vi "Configure Multipoint.vi"(5 "Sample Interval (1 Second)":dbl=1.0 format="%#.6g", 6 "Sample Source (0: Immediate)":i32(ring) items=["Immediate", "Timer"], 7 "Pretrigger Count (0)":i32 format="%#.6g", 8 "error in (no error)":errorcluster, 9 "Sample Count (1)":i32=1 format="%#.6g", 10 "Trigger Count (1)":i32=1 format="%#.6g", 11 "VISA resource name":refnum<visa-resource-name>) -> (0 "error out":errorcluster, 3 "VISA resource name out":refnum<visa-resource-name>)   [LabVIEW 2020, in "Agilent 3446X Series.lvlib"]
doc: "Configures trigger count and sample count so you can take multipoint measurements.\n\nNote: Use this VI only with other low-level VIs. The high-level VIs automatically incorporate this functionality."
uses:
  Agilent 3446X Series.lvlib
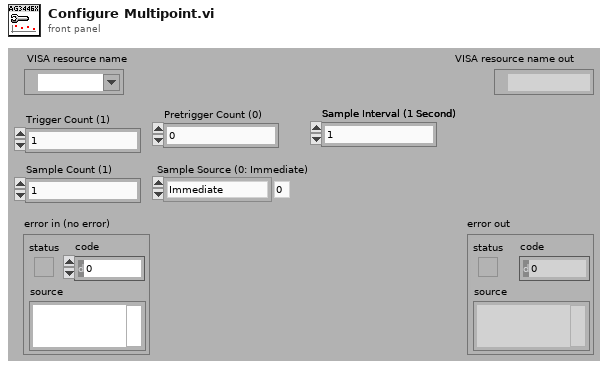
[diagram p1: front panel]
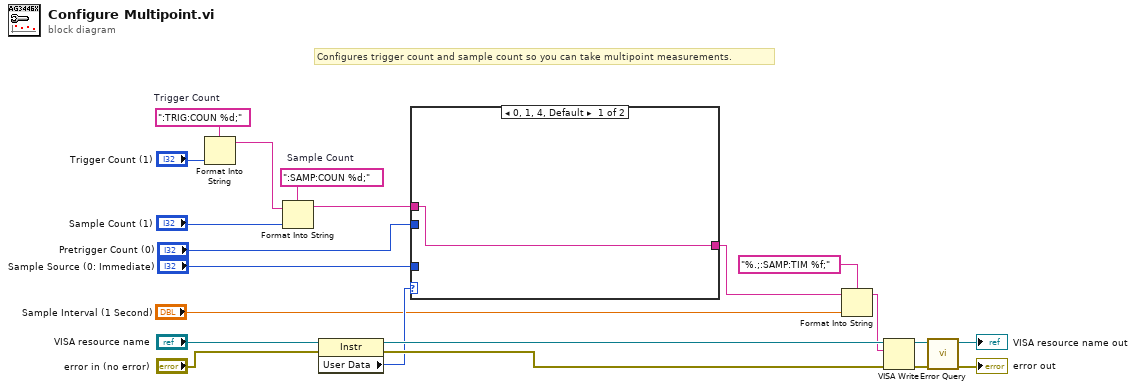
[diagram p0: block diagram]
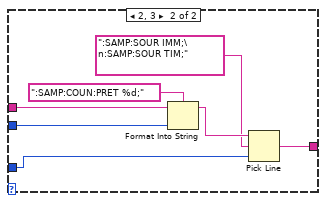
[diagram p2: hidden frame]
diagram:
  w15 = ":SAMP:COUN %d;"  # Sample Count
  w16 = ":TRIG:COUN %d;"  # Trigger Count
  # "Configures trigger count and sample count so you can take multipoint measurements."
  n1 = Format Into String(format string=w16, "Trigger Count (1)") -> (resulting string=w13:string)  [unwired: 2 in, 1 out]
  n2 = Format Into String(format string=w15, initial string=w13, "Sample Count (1)") -> (resulting string=w6:string)  [unwired: 1 in, 1 out]
  n3 = property class="Instr"(reference="VISA resource name", error in="error in (no error)") -> (reference out=w11:refnum<visa-resource-name>, error out=w10:errorcluster, "User Data"=w8:u32)
  n4 = case shown="0, 1, 4, Default" w8 {
    tunnel: w6 -> [w22 w27]
    tunnel: [w22 w25] -> w4
    tunnel: "Pretrigger Count (0)" -> [_ w29]
    tunnel: "Sample Source (0: Immediate)" -> [_ w23]
    frame 0, 1, 4, Default {
    }
    frame 2, 3 {
      n5 = Format Into String(format string=":SAMP:COUN:PRET %d;", initial string=w27, w29) -> (resulting string=w26:string)  [unwired: 1 in, 1 out]
      n6 = Pick Line(string ("")=w26, multi-line string=":SAMP:SOUR IMM;\n:SAMP:SOUR TIM;", line index=w23) -> (output string=w25:string)
    }
  }
  n7 = Format Into String(format string="%.;:SAMP:TIM %f;", initial string=w4, "Sample Interval (1 Second)") -> (resulting string=w3:string)  [unwired: 1 in, 1 out]
  n8 = VISA Write(VISA resource name=w11, write buffer=w3, error in (no error)=w10) -> (VISA resource name out=w19:refnum<visa-resource-name>, error out=w18:errorcluster)  [unwired: 1 out]
  n9 = call "Error Query.vi"("error in (no error)"=w18, "VISA resource name"=w19) -> ("error out"=→"error out":errorcluster, "VISA resource name out"=→"VISA resource name out":refnum<visa-resource-name>)  [unwired: 8 out]
